vi "TLV to TableRow.vi"(8 "error in (no error)":errorcluster, 11 "Protocol Verification Test in":refnum<class "Protocol Verification Test.lvclass">) -> (0 "error out":errorcluster, 3 "Protocol Verification Test out":refnum<class "Protocol Verification Test.lvclass">)   [LabVIEW 2017, in "Protocol Verification Test.lvlib" / "Protocol Verification Test.lvclass"]
uses:
  Protocol Verification Test.lvclass
  Protocol Verification Test.lvclass/Protocol Verification Test.ctl
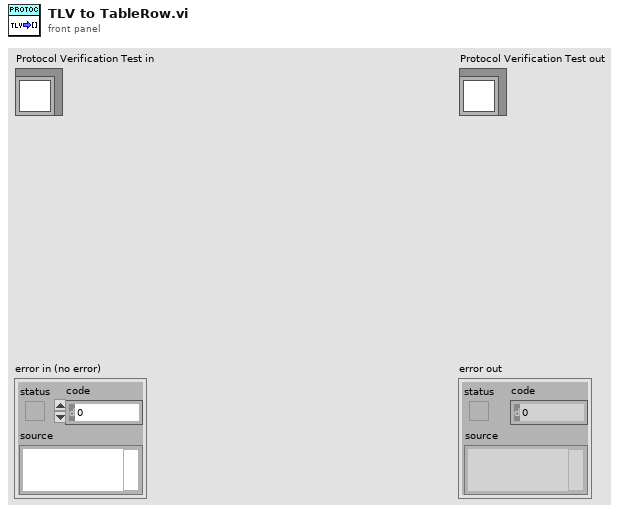
[diagram p1: front panel]
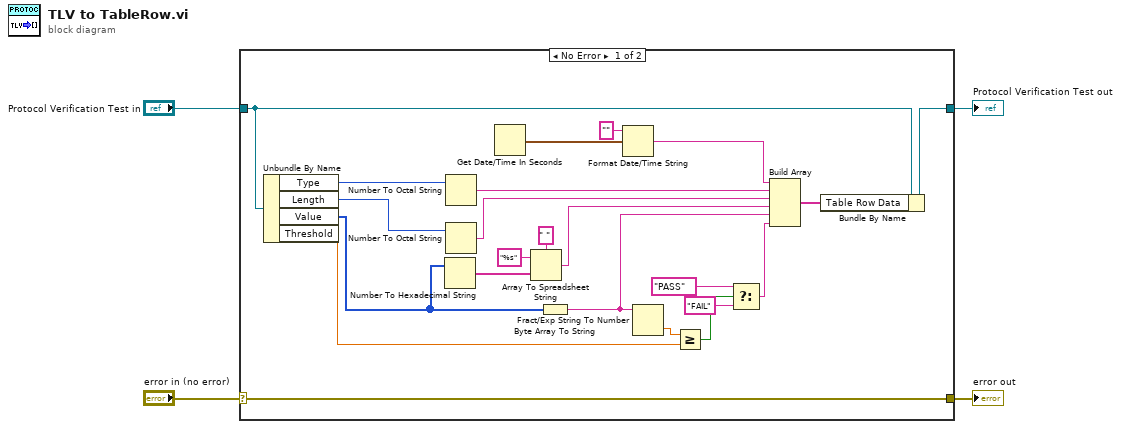
[diagram p0: block diagram]
diagram:
  n1 = case shown="No Error" "error in (no error)" {
    selector: "error in (no error)" -> [w27 w29]
    tunnel: [w27 w29] -> w3
    tunnel: [w15 w28] -> w1
    tunnel: "Protocol Verification Test in" -> [w19 w28]
    frame No Error {
      n2 = Unbundle By Name(w19) -> ("Type"=w17:u8, "Length"=w18:u8, "Value"=w6:u8[], "Threshold"=w16:dbl)
      n3 = Number To Hexadecimal String(2:w6) -> (0:w9:string[])  [unwired: 1 in]
      n4 = Number To Octal String(2:w17) -> (0:w26:string)  [unwired: 1 in]
      n5 = Number To Octal String(2:w18) -> (0:w25:string)  [unwired: 1 in]
      n6 = Get Date/Time In Seconds() -> (seconds since 1Jan1904=w13:timestamp)
      n7 = Array To Spreadsheet String(delimiter (Tab)=" ", array=w9, 3:"%s" ("format string")) -> (spreadsheet string=w5:string)
      n8 = Byte Array To String(unsigned byte array=w6) -> (string=w10:string)
      n9 = Format Date/Time String(time format string (%c)="", seconds (now)=w13) -> (date/time string=w11:string)  [unwired: 1 in]
      n10 = Fract/Exp String To Number(string=w10) -> (number=w24:dbl)  [unwired: 3 in, 1 out]
      n11 = Greater Or Equal?(x=w24, y=w16) -> (x >= y?=w23:bool)
      n12 = Select(t="PASS" ("delimiter (Tab)"), s=w23, f="FAIL") -> (s? t:f=w20:string)
      n13 = Build Array(w11, w26, w25, w5, w10, w20) -> (w14:string[])
      n14 = Bundle By Name(cluster=w19, "Table Row Data"=w14) -> (w15:refnum<class "Protocol Verification Test.lvclass">)
    }
    frame Error {
    }
  }
  "error out" <- w3
  "Protocol Verification Test out" <- w1
